vi "average data HRT.vi"(8 "error in (no error)":errorcluster, 9 "Coagulant":T2={"flocculator volume (L)"=100.0, "clarifier volume (L)"=0.0, "dose updates per HRT"=0, "target clarified turbidity (NTU)"=0.3, "Coagulant mode"=enum."manual", "Coag dose [mg/L]"=0.0, "pump mL/rev"=0.0, "clarifier flow [L/s]"=0.5, "min Coag dose [mg/L]"=0.0, "max Coag dose [mg/L]"=0.0, "Steps"=3} {"Steps" min=3 step=1; "clarifier flow [L/s]" min=0.0001 max=1.0 step=0.0001; "target clarified turbidity (NTU)" min=0.1 max=5.0 step=0.01; "dose updates per HRT" min=1 max=1000 step=1}, 10 "data input":T4, 11 "seconds since 1Jan1904":timestamp) -> (0 "error out":errorcluster, 1 "new interval":bool, 2 "total HRT":dbl, 3 "averaged data":T1)   [LabVIEW 2015]
uses:
  coag model data.ctl
  coag.ctl
  model type.ctl
  data cluster.ctl
  Sensor buffer command.ctl
panel:
  # "min"
  # "max"
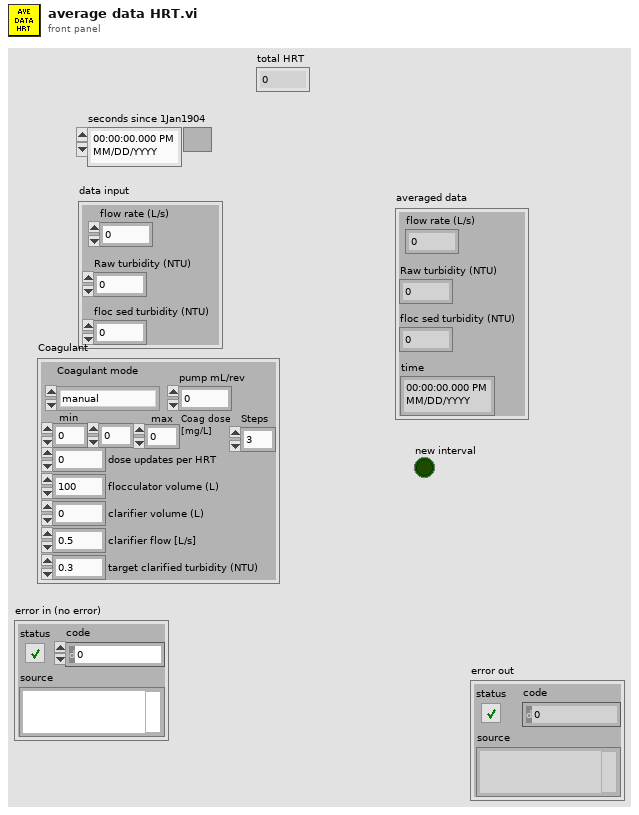
[diagram p1: front panel]
types:
  T1 = typedef "data cluster.ctl" = cluster{"floc sed turbidity (NTU)":dbl, "Raw turbidity (NTU)":dbl, "flow rate (L/s)":dbl, "time":timestamp}
  T2 = typedef "coag.ctl" = cluster{"flocculator volume (L)":dbl, "clarifier volume (L)":dbl, "dose updates per HRT":u32, "target clarified turbidity (NTU)":dbl, "Coagulant mode":T3, "Coag dose [mg/L]":dbl, "pump mL/rev":dbl, "clarifier flow [L/s]":dbl, "min Coag dose [mg/L]":dbl, "max Coag dose [mg/L]":dbl, "Steps":u16}
  T3 = typedef "model type.ctl" = enum16{"manual", "ramp", "simple corrector", "linear regression"}
  T4 = typedef "coag model data.ctl" = cluster{"flow rate (L/s)":dbl, "Raw turbidity (NTU)":dbl, "floc sed turbidity (NTU)":dbl}
  T5 = typedef "Sensor buffer command.ctl" = enum16{"set buffer size", "write", "refill buffer", "read recent", "read all", "clear"}
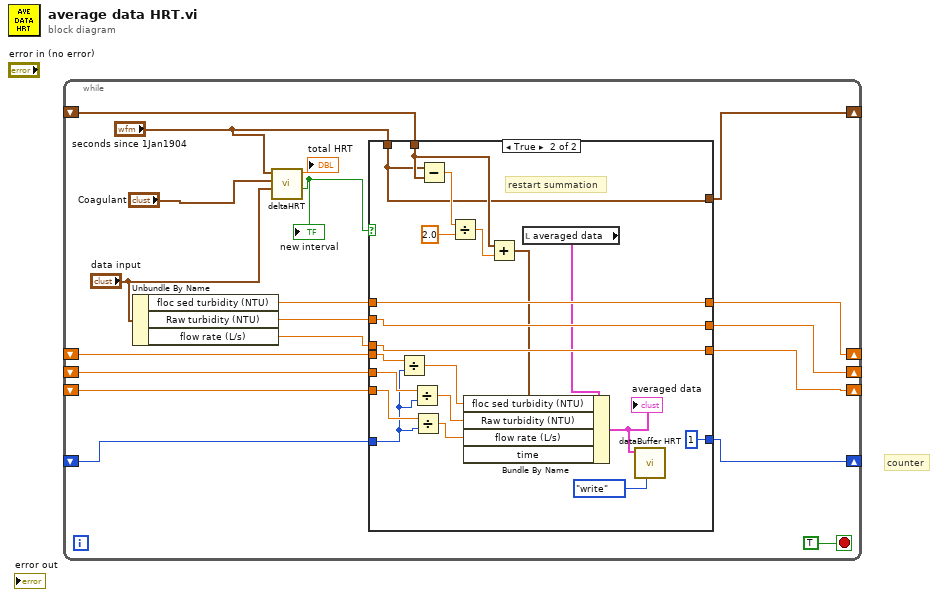
[diagram p0: block diagram]
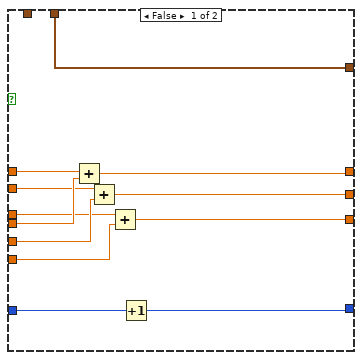
[diagram p2: hidden frame]
diagram:
  # "counter"
  n1 = while {
    shift-right: [w16] -> _
    shift-left: _ -> [w15]
    shift-right: [w18] -> _
    shift-left: _ -> [w17]
    shift-right: [w14] -> _
    shift-left: _ -> [w12]
    shift-right: [w10] -> _
    shift-left: _ -> [w9]
    shift-right: [w6] -> _
    shift-left: _ -> [w7]
    stop <- TRUE stop-if-true
    n2 = Unbundle By Name("data input") -> ("floc sed turbidity (NTU)"=w13:dbl, "Raw turbidity (NTU)"=w11:dbl, "flow rate (L/s)"=w8:dbl)
    n3 = call "deltaHRT.vi"("data input"="data input", "Coagulant"="Coagulant", "seconds since 1Jan1904"="seconds since 1Jan1904") -> ("new interval"=w4:bool, "total HRT"=→"total HRT":dbl)  [unwired: 6 in, 1 out]
    "new interval" <- w4
    n4 = case shown="True" w4 {
      tunnel: [w30 1] -> w18
      tunnel: w17 -> [w31 w42]
      tunnel: [w29 w34] -> w16
      tunnel: "seconds since 1Jan1904" -> [_ w34]
      tunnel: w15 -> [w29 w35]
      tunnel: [w26 w50] -> w14
      tunnel: w13 -> [w27 w50]
      tunnel: w12 -> [w28 w47]
      tunnel: w11 -> [w25 w49]
      tunnel: [w23 w49] -> w10
      tunnel: w9 -> [w24 w45]
      tunnel: w8 -> [w22 w48]
      tunnel: w7 -> [w21 w43]
      tunnel: [w20 w48] -> w6
      frame False {
        n5 = Add(x=w27, y=w28) -> (x+y=w26:dbl)
        n6 = Add(x=w25, y=w24) -> (x+y=w23:dbl)
        n7 = Add(x=w22, y=w21) -> (x+y=w20:dbl)
        n8 = Increment(x=w31) -> (x+1=w30:i32)
      }
      frame True {
        # "restart summation"
        n9 = Divide(x=w47, y=w42) -> (x/y=w46:dbl)
        n10 = Divide(x=w45, y=w42) -> (x/y=w44:dbl)
        n11 = Divide(x=w43, y=w42) -> (x/y=w41:dbl)
        n12 = Subtract(x=w34, y=w35) -> (x-y=w38:dbl)
        n13 = Divide(x=w38, y=2.0) -> (x/y=w37:dbl)
        n14 = Add(x=w35, y=w37) -> (x+y=w36:timestamp)
        n15 = local read "averaged data"() -> (w40:T1)
        n16 = Bundle By Name(cluster=w40, "floc sed turbidity (NTU)"=w46, "Raw turbidity (NTU)"=w44, "flow rate (L/s)"=w41, "time"=w36) -> (w33:T1)
        "averaged data" <- w33
        n17 = call "dataBuffer HRT.vi"("command"=Sensor_buffer_command."write", "averaged data"=w33) -> ()  [unwired: 6 in, 4 out]
      }
    }
  }
